vi "Set Type.vi"(10 "Type":refnum<class "Type.lvclass">, 11 "TextPanel in":refnum<class "TextPanel.lvclass">) -> (3 "TextPanel out":refnum<class "TextPanel.lvclass">)   [LabVIEW 2020, in "Conditum-Tools.lvlib" / "TextPanel.lvclass"]
uses:
  TextPanel.lvclass
  Conditum-Clone/Columns/Type/Type.lvclass
  TextPanel.lvclass/TextPanel.ctl
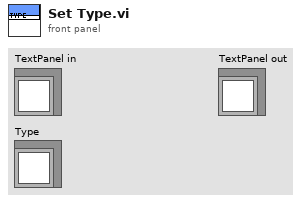
[diagram p1: front panel]
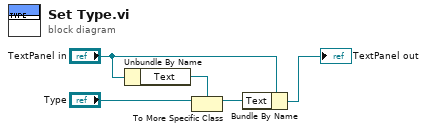
[diagram p0: block diagram]
diagram:
  n1 = Unbundle By Name("TextPanel in") -> ("Text"=w4:refnum<class "Text.lvclass">)
  n2 = To More Specific Class(target class=w4, reference="Type") -> (specific class reference=w5:refnum<class "Text.lvclass">)  [unwired: 1 in, 1 out]
  n3 = Bundle By Name(cluster="TextPanel in", "Text"=w5) -> (→"TextPanel out":refnum<class "TextPanel.lvclass">)
